vi "Table_ReadDataAndUpdateTable.vi"(6 "Enable Limits":bool, 7 "Limit Settings":variant, 8 "error in (no error)":errorcluster, 9 "Data":string[][](array[string]), 10 "Listbox Ref":refnum<vi>, 11 "WorkspaceManager":T1) -> (0 "error out":errorcluster, 1 "Data Out":string[][](array[string]), 2 "Listbox Ref Out":refnum<vi>, 5 "Limit Settings Out":variant)   [LabVIEW 2012, in "TableSupportLib.lvlib"]
uses:
  TableSupportLib.lvlib
  <vilib>/NI Veristand/Execution/Workspace/WorkspaceAPI.ctl
  NationalInstruments.VeriStand.ClientAPI
  <vilib>/Utility/miscctls.llb/LVRowAndColumnTypeDef.ctl
  Table_LimitSettings.ctl
  <vilib>/NI Veristand/Execution/Workspace/NI VeriStand - Get Multiple Channel Values.vi
  Table_Globals.vi
  <vilib>/NI Veristand/Execution/Workspace/NI_VS Workspace ExecutionAPI.lvlib
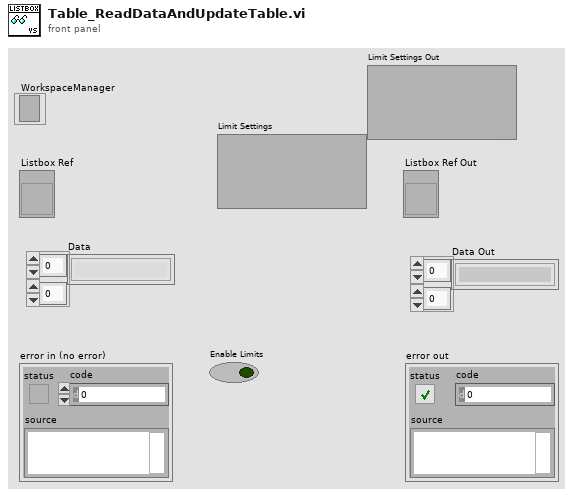
[diagram p1: front panel]
types:
  T1 = typedef "NI_VS Workspace ExecutionAPI.lvlib/WorkspaceAPI.ctl" = refnum<k24>
  T2 = typedef "TableSupportLib.lvlib/Table_LimitSettings.ctl" = cluster{"High":dbl, "High Warning":dbl, "Low Warning":dbl, "Low":dbl}
  T3 = typedef "LVRowAndColumnTypeDef.ctl" = cluster{"Row":i32, "Column":i32}
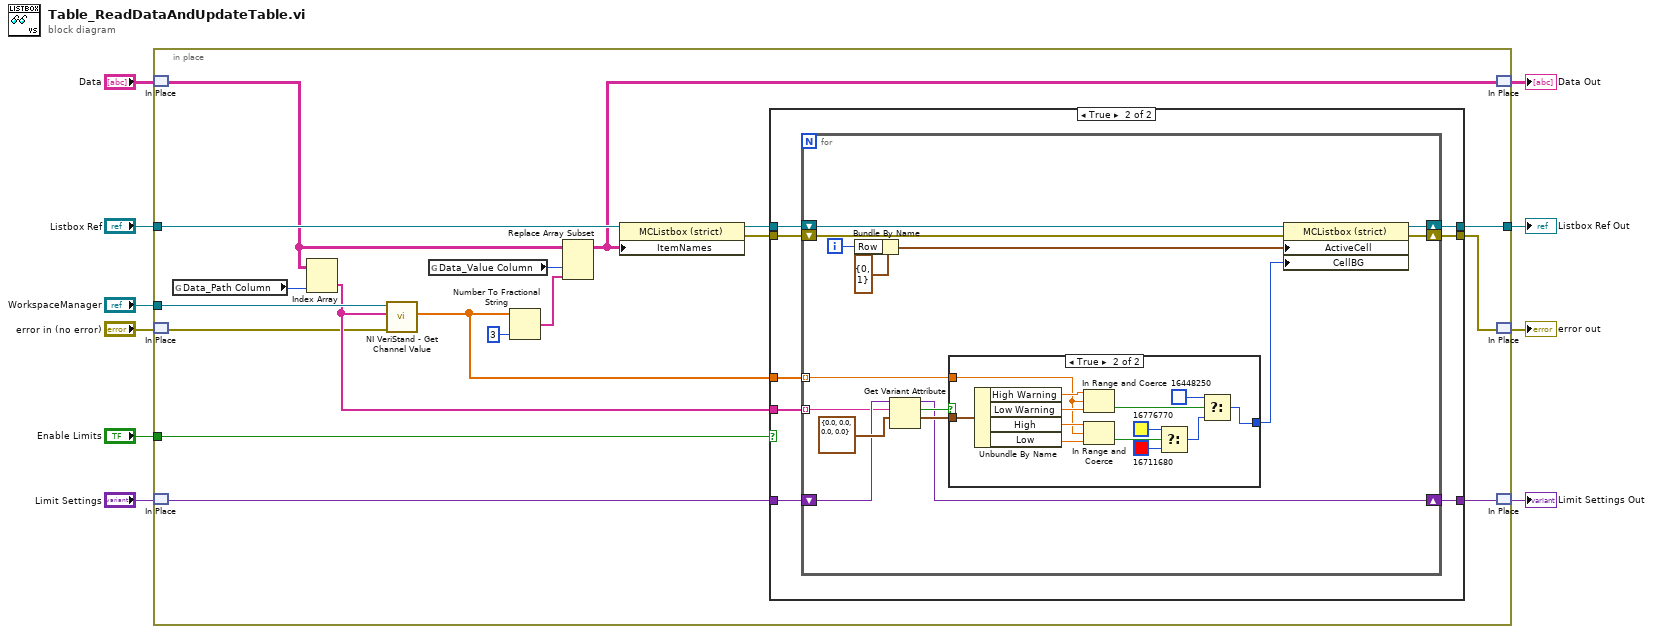
[diagram p0: block diagram]
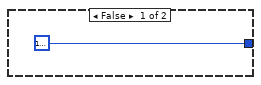
[diagram p3: hidden frame]
diagram:
  n1 = in-place {
    in-place-border: "WorkspaceManager" -> [w28]
    in-place-border: "Listbox Ref" -> [w27]
    in-place-border: [w24] -> w8
    in-place-border: "Enable Limits" -> [w23]
    n2 = in-place-match #1("Data") -> (w14:string[][])
    n3 = in-place-match #2("error in (no error)") -> (w12:errorcluster)
    n4 = in-place-match #3("Limit Settings") -> (w16:variant)
    n5 = global read "Table_Globals.vi" "Data_Path Column"() -> (w19:i32)
    n6 = Index Array(array=w14, index (col)=w19) -> (element=w22:string[])  [unwired: 1 in]
    n7 = call-poly <vilib>:"NI VeriStand - Get Channel Value.vi"("error in (no error)"=w12, "Channels"=w22, "WorkspaceManager in"=w28) -> ("Values"=w21:dbl[])  [unwired: 6 in, 2 out]
    n8 = global read "Table_Globals.vi" "Data_Value Column"() -> (w20:i32)
    n9 = Number To Fractional String(number=w21, precision (6)=i16 3) -> (F-format string=w17:string[])  [unwired: 2 in]
    n10 = Replace Array Subset(array=w14, new element=w17, index (col)=w20) -> (w13:string[][])  [unwired: 1 in]
    n11 = property on="Property Node" class="MCListbox (strict)"(reference=w27, "ItemNames"=w13) -> (reference out=w25:refnum<vi>, error out=w26:errorcluster)  [unwired: 1 in]
    n12 = case shown="True" w23 {
      tunnel: w26 -> [w31 w39]
      tunnel: [w31 w38] -> w11
      tunnel: w25 -> [w30 w37]
      tunnel: [w30 w36] -> w24
      tunnel: w16 -> [w29 w35]
      tunnel: w22 -> [_ w34]
      tunnel: w21 -> [_ w33]
      tunnel: [w29 w32] -> w15
      frame False {
      }
      frame True {
        n13 = for {
          shift-right: [w49] -> w36
          shift-left: w37 -> [w50]
          shift-right: [w48] -> w38
          shift-left: w39 -> [w51]
          tunnel: w34 -> [w43] mode=indexing
          tunnel: w33 -> [w42] mode=indexing
          shift-right: [w40] -> w32
          shift-left: w35 -> [w44]
          i -> [w53]
          n14 = Bundle By Name(cluster=T3 {"Row"=0, "Column"=1} ("Active Cell:Active Cell"), "Row"=w53) -> (w52:T3)
          n15 = Get Variant Attribute(Variant=w44, name=w43, default value (empty Variant)=T2 {"High"=0.0, "High Warning"=0.0, "Low Warning"=0.0, "Low"=0.0} ("Limits")) -> (duplicate Variant=w40:variant, found=w45:bool, value=w46:T2)  [unwired: 1 in, 1 out]
          n16 = case shown="True" w45 {
            tunnel: w46 -> [_ w68]
            tunnel: [u32 16777216 w60] -> w41
            tunnel: w42 -> [_ w63]
            frame False {
            }
            frame True {
              n17 = Unbundle By Name(w68) -> ("High Warning"=w67:dbl, "Low Warning"=w66:dbl, "High"=w65:dbl, "Low"=w64:dbl)
              n18 = In Range and Coerce(upper limit=w67, x=w63, lower limit=w66) -> (In Range?=w62:bool)  [unwired: 1 out]
              n19 = In Range and Coerce(upper limit=w65, x=w63, lower limit=w64) -> (In Range?=w59:bool)  [unwired: 1 out]
              n20 = Select(t=u32 16776770, s=w59, f=u32 16711680) -> (s? t:f=w56:u32)
              n21 = Select(t=u32 16448250, s=w62, f=w56) -> (s? t:f=w60:u32)
            }
          }
          n22 = property on="Property Node" class="MCListbox (strict)"(reference=w50, error in=w51, "ActiveCell"=w52, "CellBG"=w41) -> (reference out=w49:refnum<vi>, error out=w48:errorcluster)
        }
      }
    }
    n23 = in-place-match #1(w13) -> (→"Data Out":string[][])
    n24 = in-place-match #2(w11) -> (→"error out":errorcluster)
    n25 = in-place-match #3(w15) -> (→"Limit Settings Out":variant)
  }
  "Listbox Ref Out" <- w8
